vi "Check File Extension.vi"(11 "path in":path) -> (3 "path out":path)   [LabVIEW 2014, in "C Header Generator.lvlib"]
uses:
  C Header Generator.lvlib
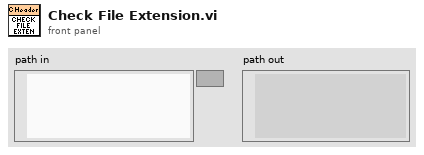
[diagram p1: front panel]
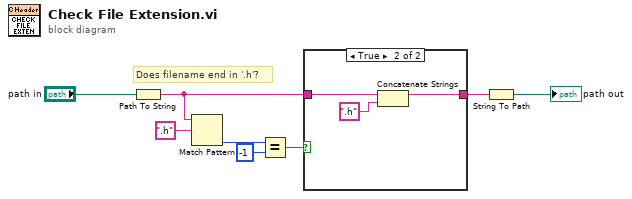
[diagram p0: block diagram]
diagram:
  # "Does filename end in '.h'?"
  n1 = Path To String(path="path in") -> (string=w3:string)
  n2 = Match Pattern(string=w3, regular expression=".h") -> (offset past match=w6:i32)  [unwired: 1 in, 3 out]
  n3 = Equal?(x=w6, y=-1) -> (x = y?=w4:bool)
  n4 = case shown="True" w4 {
    tunnel: w3 -> [w9 w12]
    tunnel: [w9 w10] -> w2
    frame False {
    }
    frame True {
      n5 = Concatenate Strings(w12, ".h") -> (w10:string)
    }
  }
  n6 = String To Path(string=w2) -> (path=→"path out":path)
